vi "TREE_Get Siblings__jki_lib_tree_control -- VI Tester.vi"(0 "Tree Reference In":refnum<vi>, 2 "Input Tag (Current)":string, 5 "error in (no error)":errorcluster) -> (14 "Tree Reference Out":refnum<vi>, 16 "Sibling Tags":string[](array[string]), 19 "error out":errorcluster)   [LabVIEW 2011]
doc: "Retrieves a 1-D array of tags of all items in the tree that have the same parent and deletes the requested tag giving all siblings of an item. Uses the currently selected item if the tag input is unwired."
panel:
  # "VI INPUTS"
  # "VI OUTPUTS"
  # "***TREE_Get Siblings.vi***\n\n***Retrieves a 1-D array of tags of all items in the tree that have the same parent*** \n\nPlease visit    http://forums.lavag.org/forums.html   and   http://www.OpenG.org\nto learn about the Open Source LabVIEW software movement.\n\nNOTICE -- YOU MUST LEAVE THIS NOTICE IN PLACE.  PER THE TERMS OF THE LICENSE BELOW, YOU MAY SUBLICENSE THIS SOFTWARE \nIN ANY WAY THAT DOES NOT CONFLICT WITH THIS LICENSE.\n\n### BSD License (http://www.opensource.org/licenses/bsd-license.php) Begin ###\n \nCopyright (c) 2007, Norman J. Kirchner, Jr <NJKirchner@hotmail.com>\n\nAll rights reserved.\n\nRedistribution and use in source and binary forms, with or without modification, are permitted provided that the following conditions are met:\n\n    * Redistributions of source code must retain the above copyright notice, this list of conditions and the following disclaimer.\n    * Redistributions in binary form must reproduce the above copyright notice, this list of conditions and the following disclaimer in the \n       documentation and/or other materials provided with the distribution.\n    * Neither the name of SciWare, James Kring, Inc., nor the names of its contributors may be used to endorse or promote products derived \n       from this software without specific prior written permission.\n\nTHIS SOFTWARE IS PROVIDED BY THE COPYRIGHT HOLDERS AND CONTRIBUTORS \"AS IS\" AND ANY EXPRESS OR IMPLIED WARRANTIES, \nINCLUDING, BUT NOT LIMITED TO, THE IMPLIED WARRANTIES OF MERCHANTABILITY AND FITNESS FOR A PARTICULAR PURPOSE ARE \nDISCLAIMED. IN NO EVENT SHALL THE COPYRIGHT OWNER OR CONTRIBUTORS BE LIABLE FOR ANY DIRECT, INDIRECT, INCIDENTAL,\n SPECIAL, EXEMPLARY, OR CONSEQUENTIAL DAMAGES (INCLUDING, BUT NOT LIMITED TO, PROCUREMENT OF SUBSTITUTE GOODS OR \nSERVICES; LOSS OF USE, DATA, OR PROFITS; OR BUSINESS INTERRUPTION) HOWEVER CAUSED AND ON ANY THEORY OF LIABILITY, \nWHETHER IN CONTRACT, STRICT LIABILITY, OR TORT (INCLUDING NEGLIGENCE OR OTHERWISE) ARISING IN ANY WAY OUT OF THE USE \nOF THIS SOFTWARE, EVEN IF ADVISED OF THE POSSIBILITY OF SUCH DAMAGE.\n\n### BSD License End ###"
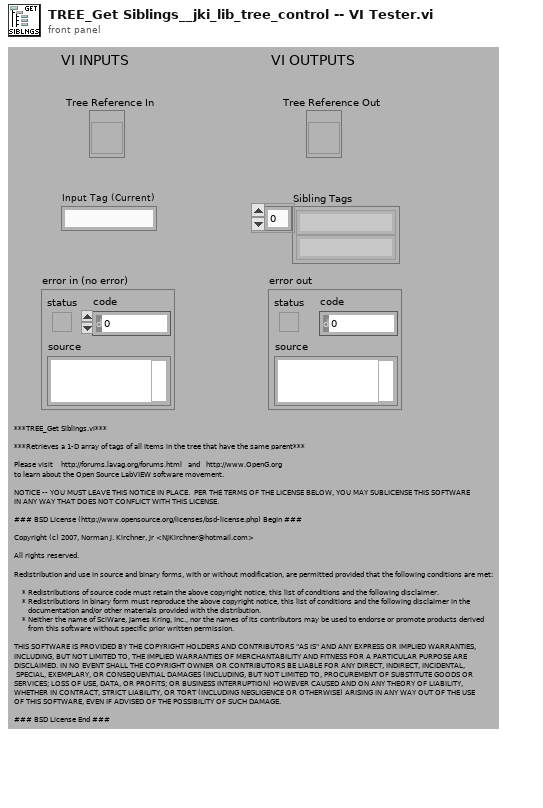
[diagram p1: front panel]
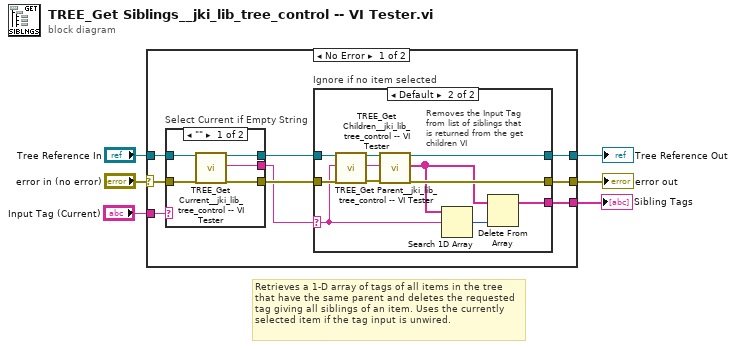
[diagram p0: block diagram]
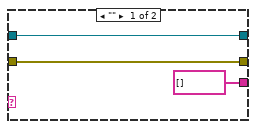
[diagram p2: hidden frame]
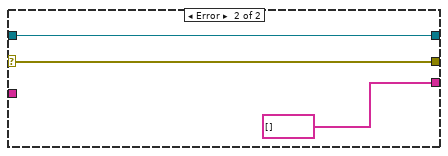
[diagram p4: hidden frame]
diagram:
  # "Retrieves a 1-D array of tags of all items in the tree that have the same parent and deletes the requested tag giving all siblings of an item. Uses the currently selected item if the tag input is unwired."
  n1 = case shown="No Error" "error in (no error)" {
    selector: "error in (no error)" -> [w10 w39]
    tunnel: "Tree Reference In" -> [w12 w40]
    tunnel: "Input Tag (Current)" -> [w8 _]
    tunnel: [w15 w40] -> w4
    tunnel: [w13 string[] []] -> w3
    tunnel: [w14 w39] -> w2
    frame No Error {
      n2 = case "Select Current if Empty String" shown="\"\"" w8 {
        selector: w8 -> [_ w35]
        tunnel: [w33 w37] -> w11
        tunnel: w12 -> [w34 w37]
        tunnel: [w32 w36] -> w9
        tunnel: w10 -> [w31 w36]
        tunnel: [w30 w35] -> w7
        frame "" {
          n3 = call "TREE_Get Current__jki_lib_tree_control -- VI Tester.vi"("Tree Reference In"=w34, "error in (no error)"=w31) -> ("Tree Reference Out"=w33:refnum<vi>, "Current Tag"=w30:string, "error out"=w32:errorcluster)  [unwired: 14 in, 1 out]
        }
        frame Default {
        }
      }
      n4 = case "Ignore if no item selected" shown="Default" w7 {
        selector: w7 -> [_ w19]
        tunnel: [w18 w26] -> w15
        tunnel: [w17 w25] -> w14
        tunnel: [string[] [] ("Children Tags") w23] -> w13
        tunnel: w11 -> [w18 w22]
        tunnel: w9 -> [w17 w21]
        frame "" {
        }
        frame Default {
          # "Removes the Input Tag from list of siblings that is returned from the get children VI"
          n5 = call "TREE_Get Parent__jki_lib_tree_control -- VI Tester.vi"("Tree Reference In"=w22, "Child Tag (Current)"=w19, "error in (no error)"=w21) -> ("Tree Reference Out"=w29:refnum<vi>, "Parent Tag"=w28:string, "error out"=w27:errorcluster)  [unwired: 13 in, 1 out]
          n6 = call "TREE_Get Children__jki_lib_tree_control -- VI Tester.vi"("Tree Reference In"=w29, "Parent Tag"=w28, "error in (no error)"=w27) -> ("Tree Reference Out"=w26:refnum<vi>, "Children Tags"=w20:string[], "error out"=w25:errorcluster)  [unwired: 14 in]
          n7 = Search 1D Array(1D array=w20, element=w19) -> (index of element=w24:i32)  [unwired: 1 in]
          n8 = Delete From Array(array=w20, index=w24) -> (array with subset deleted=w23:string[])  [unwired: 1 in, 1 out]
        }
      }
    }
    frame Error {
    }
  }
  "Sibling Tags" <- w3
  "Tree Reference Out" <- w4
  "error out" <- w2
